vi "Write OCP Level.vi"(8 "error in":errorcluster, 10 "OCP Level":dbl, 11 "Electronic Load in":refnum<class "Electronic Load.lvclass">) -> (0 "error out":errorcluster, 3 "Electronic Load out":refnum<class "Electronic Load.lvclass">)   [LabVIEW 2019, in "Electronic Load.lvlib" / "Electronic Load.lvclass"]
uses:
  Library/Electronic Load.lvclass
  C:/Users/Public/Documents/Development/builds/Engine/Monitored Actor.lvlibp/Monitored Actor/Monitored Actor/Monitored Actor.lvclass
  C:/Users/Public/Documents/Development/builds/Instruments/Instruments.lvlibp/Library/Instruments.lvclass
  Library/Electronic Load.lvclass/Electronic Load.ctl
  builds/Engine/Monitored Actor.lvlibp/Monitored Actor/Monitored Actor/Read Actor Label.vi
  builds/Instruments/Instruments.lvlibp/Private/Polymorphic/Integers/Event from DBL.vi
  builds/Instruments/Instruments.lvlibp/Accessors/Command with Logging.vi
  builds/Instruments/Instruments.lvlibp/Library/Instruments.lvclass
  builds/Instruments/Instruments.lvlibp
  builds/Engine/Engine.lvlibp/Project/Engine.lvclass
  C:/Users/Public/Documents/Development/builds/Engine/Engine.lvlibp/Project/Engine.lvclass
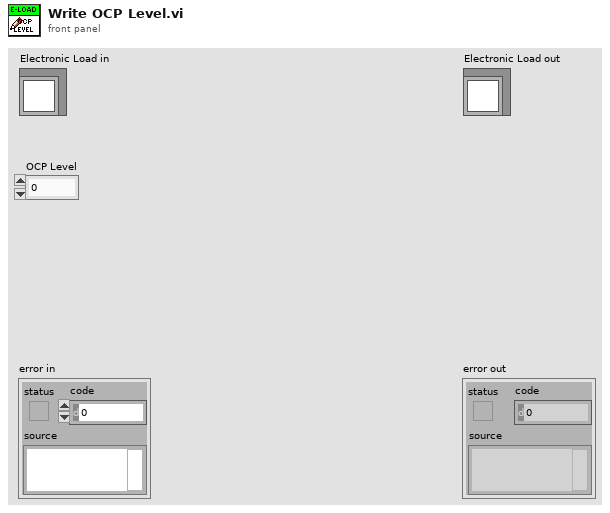
[diagram p1: front panel]
types:
  T1 = typedef "Electronic Load.lvlib/Electronic Load.lvclass/OCP Settings.ctl" = cluster{"OCP_Enabled":bool, "OCP Level":dbl, "OCP Delay":dbl}
  T2 = typedef "Electronic Load.lvlib/Electronic Load.lvclass/Limits.ctl" = cluster{"Max Voltage":dbl, "Min Voltage":dbl, "Max Current":dbl, "Min Current":dbl}
  T3 = cluster{"Timestamp":timestamp, "Description":string, "Data":string}
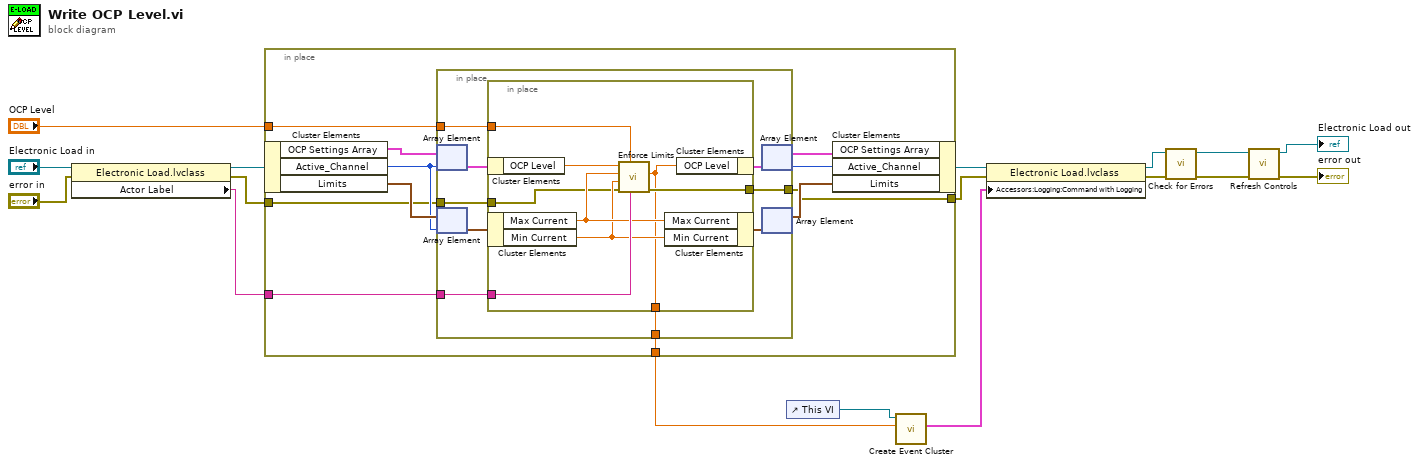
[diagram p0: block diagram]
diagram:
  n1 = property class="Electronic Load.lvclass"(reference="Electronic Load in", error in="error in") -> (reference out=w12:refnum<class "Electronic Load.lvclass">, error out=w10:errorcluster, "Actor Label"=w11:string)
  n2 = in-place {
    in-place-border: "OCP Level" -> [w25]
    in-place-border: w11 -> [w24]
    in-place-border: w10 -> [w20]
    in-place-border: [w19] -> w9
    in-place-border: [w18] -> w7
    n3 = in-place-cluster #1(w12) -> ("OCP Settings Array"=w28:T1[], "Active_Channel"=w22:u32, "Limits"=w23:T2[])
    n4 = in-place {
      in-place-border: w25 -> [w35]
      in-place-border: w24 -> [w34]
      in-place-border: w20 -> [w31]
      in-place-border: [w30] -> w19
      in-place-border: [w29] -> w18
      n5 = in-place-array #2(w28, w22) -> (w37:T1)
      n6 = in-place-array #3(w23, w22) -> (w33:T2)
      n7 = in-place {
        in-place-border: w35 -> [w44]
        in-place-border: w34 -> [w43]
        in-place-border: w31 -> [w40]
        in-place-border: [w39] -> w30
        in-place-border: [w38] -> w29
        n8 = in-place-cluster #4(w37) -> ("OCP Level"=w45:dbl)
        n9 = in-place-cluster #5(w33) -> ("Max Current"=w42:dbl, "Min Current"=w41:dbl)
        n10 = call "Enforce Limits.vi"("Device"=w43, "Setpoint"=w44, "error in"=w40, "Minimum"=w41, "Maximum"=w42, "Previous"=w45) -> ("error out"=w39:errorcluster, "Protected Setpoint"=w38:dbl)  [unwired: 4 in]
        n11 = in-place-cluster #5("Max Current"=w42, "Min Current"=w41) -> (w32:T2)
        n12 = in-place-cluster #4("OCP Level"=w38) -> (w36:T1)
      }
      n13 = in-place-array #2(w36) -> (w27:T1[], w26:i32)
      n14 = in-place-array #3(w32) -> (w21:T2[])  [unwired: 1 out]
    }
    n15 = in-place-cluster #1("OCP Settings Array"=w27, "Active_Channel"=w26, "Limits"=w21) -> (w15:refnum<class "Electronic Load.lvclass">)
  }
  n16 = control-ref of="This VI"() -> (w17:refnum<vi>)
  n17 = call-poly "Create Event Cluster.vi"("Value"=w7, "VI Refnum"=w17) -> ("Event Data"=w14:T3)  [unwired: 9 in]
  n18 = property class="Electronic Load.lvclass"(reference=w15, error in=w9, "Accessors:Logging:Command with Logging"=w14) -> (reference out=w5:refnum<class "Electronic Load.lvclass">, error out=w6:errorcluster)
  n19 = call "Check for Errors.vi"("error in"=w6, "Engine in"=w5) -> ("error out"=w4:errorcluster, "Engine out"=w3:refnum<class "Electronic Load.lvclass">)  [unwired: 8 in]
  n20 = call "Refresh Controls.vi"("error in"=w4, "Electronic Load in"=w3) -> ("error out"=→"error out":errorcluster, "Electronic Load out"=→"Electronic Load out":refnum<class "Electronic Load.lvclass">)  [unwired: 8 in]
